vi "Open_Turret_PIDFs.vi"() -> (6 "output cluster":T1)   [LabVIEW 2019]
uses:
  <vilib>/Utility/file.llb/Read Delimited Spreadsheet (string).vi
panel:
  in  "Cluster":T1
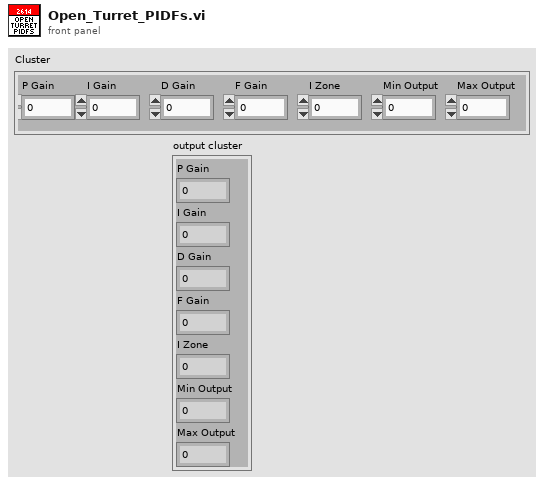
[diagram p1: front panel]
types:
  T1 = cluster{"P Gain":dbl, "I Gain":dbl, "D Gain":dbl, "F Gain":dbl, "I Zone":dbl, "Min Output":dbl, "Max Output":dbl}
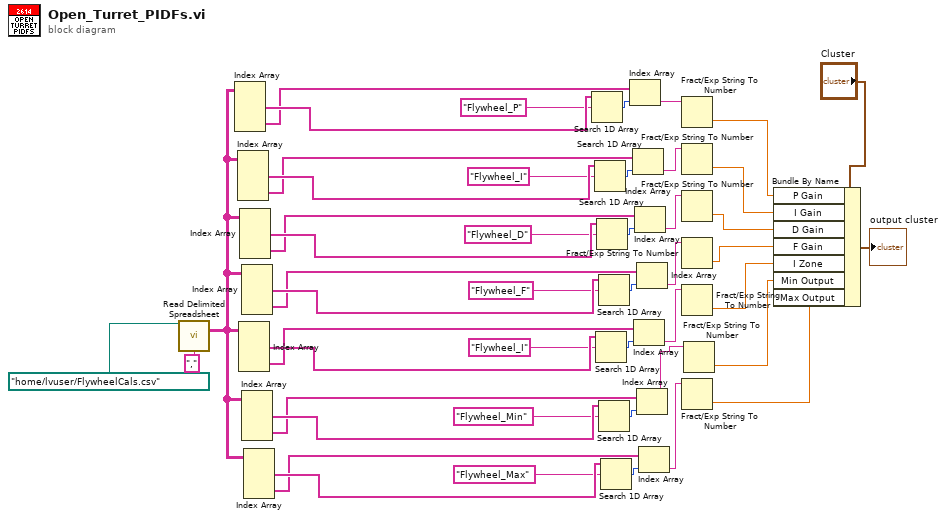
[diagram p0: block diagram]
diagram:
  n1 = call-poly <vilib>:"Read Delimited Spreadsheet.vi"("file path (dialog if empty)"=path "/home/lvuser/FlywheelCals.csv", "delimiter (\\t)"="," ("delimiter (\\t)")) -> ("all rows"=w10:string[][])  [unwired: 8 in, 5 out]
  n2 = Index Array(array=w10) -> (element #1=w30:string[], element #2=w29:string[])  [unwired: 4 in]
  n3 = Index Array(array=w10) -> (element #1=w25:string[], element #2=w24:string[])  [unwired: 4 in]
  n4 = Index Array(array=w10) -> (element #1=w45:string[], element #2=w44:string[])  [unwired: 4 in]
  n5 = Index Array(array=w10) -> (element #1=w20:string[], element #2=w19:string[])  [unwired: 4 in]
  n6 = Index Array(array=w10) -> (element #1=w15:string[], element #2=w14:string[])  [unwired: 4 in]
  n7 = Index Array(array=w10) -> (element #1=w40:string[], element #2=w39:string[])  [unwired: 4 in]
  n8 = Index Array(array=w10) -> (element #1=w35:string[], element #2=w34:string[])  [unwired: 4 in]
  n9 = Search 1D Array(1D array=w30, element="Flywheel_P") -> (index of element=w28:i32)  [unwired: 1 in]
  n10 = Search 1D Array(1D array=w25, element="Flywheel_I") -> (index of element=w23:i32)  [unwired: 1 in]
  n11 = Search 1D Array(1D array=w45, element="Flywheel_I") -> (index of element=w43:i32)  [unwired: 1 in]
  n12 = Search 1D Array(1D array=w20, element="Flywheel_D") -> (index of element=w18:i32)  [unwired: 1 in]
  n13 = Search 1D Array(1D array=w15, element="Flywheel_F") -> (index of element=w13:i32)  [unwired: 1 in]
  n14 = Search 1D Array(1D array=w40, element="Flywheel_Min") -> (index of element=w38:i32)  [unwired: 1 in]
  n15 = Search 1D Array(1D array=w35, element="Flywheel_Max") -> (index of element=w33:i32)  [unwired: 1 in]
  n16 = Index Array(array=w29, index=w28) -> (element=w26:string)
  n17 = Index Array(array=w24, index=w23) -> (element=w21:string)
  n18 = Index Array(array=w44, index=w43) -> (element=w41:string)
  n19 = Index Array(array=w19, index=w18) -> (element=w16:string)
  n20 = Index Array(array=w14, index=w13) -> (element=w11:string)
  n21 = Index Array(array=w39, index=w38) -> (element=w36:string)
  n22 = Index Array(array=w34, index=w33) -> (element=w31:string)
  n23 = Fract/Exp String To Number(string=w26) -> (number=w8:dbl)  [unwired: 3 in, 1 out]
  n24 = Fract/Exp String To Number(string=w21) -> (number=w7:dbl)  [unwired: 3 in, 1 out]
  n25 = Fract/Exp String To Number(string=w16) -> (number=w6:dbl)  [unwired: 3 in, 1 out]
  n26 = Fract/Exp String To Number(string=w11) -> (number=w5:dbl)  [unwired: 3 in, 1 out]
  n27 = Fract/Exp String To Number(string=w41) -> (number=w4:dbl)  [unwired: 3 in, 1 out]
  n28 = Fract/Exp String To Number(string=w31) -> (number=w2:dbl)  [unwired: 3 in, 1 out]
  n29 = Fract/Exp String To Number(string=w36) -> (number=w3:dbl)  [unwired: 3 in, 1 out]
  n30 = Bundle By Name(cluster="Cluster", "P Gain"=w8, "I Gain"=w7, "D Gain"=w6, "F Gain"=w5, "I Zone"=w4, "Min Output"=w3, "Max Output"=w2) -> (→"output cluster":T1)
